vi "AutoSequencer.vi"(2 "Reinit Sequencer":bool, 7 "Auto Cluster In":T1) -> (8 "Auto Cluster Out":T1)   [LabVIEW 2020]
doc: "This VI manages the autonomous sequence. The drive base and manipulator sequencers operate in parallel. Autonomous plays are written as text files and uploaded to the roboRIO via FileZilla. The appropriate play is slected prior to the match via the FRC 4265 Dashboard. For each sequencer, each step is composed of a command and a parameter string of arbitrary length. Error checking and handling is supported. An autonomous test mode (for simulating autonomous plays on the robot cart) is supported. Status updates are sent to the FRC Driver Station and the FRC 4265 Dashboard throughout autonomous. Note that the autonomous sequencer may be also active during the begining of TeleOperated mode, as determined by the MasterRobotModeController.vi."
uses:
  GlobalPoseAndTargeting.vi
  GlobalDriverStationData.vi
  GlobalAutonomous.vi
panel:
  in  "Type Def":T1
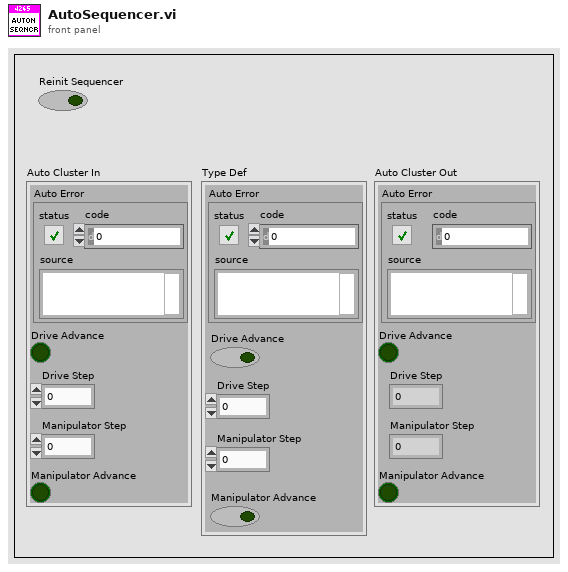
[diagram p1: front panel]
types:
  T1 = cluster{"Auto Error":errorcluster, "Drive Advance":bool, "Drive Step":i32, "Manipulator Step":i32, "Manipulator Advance":bool}
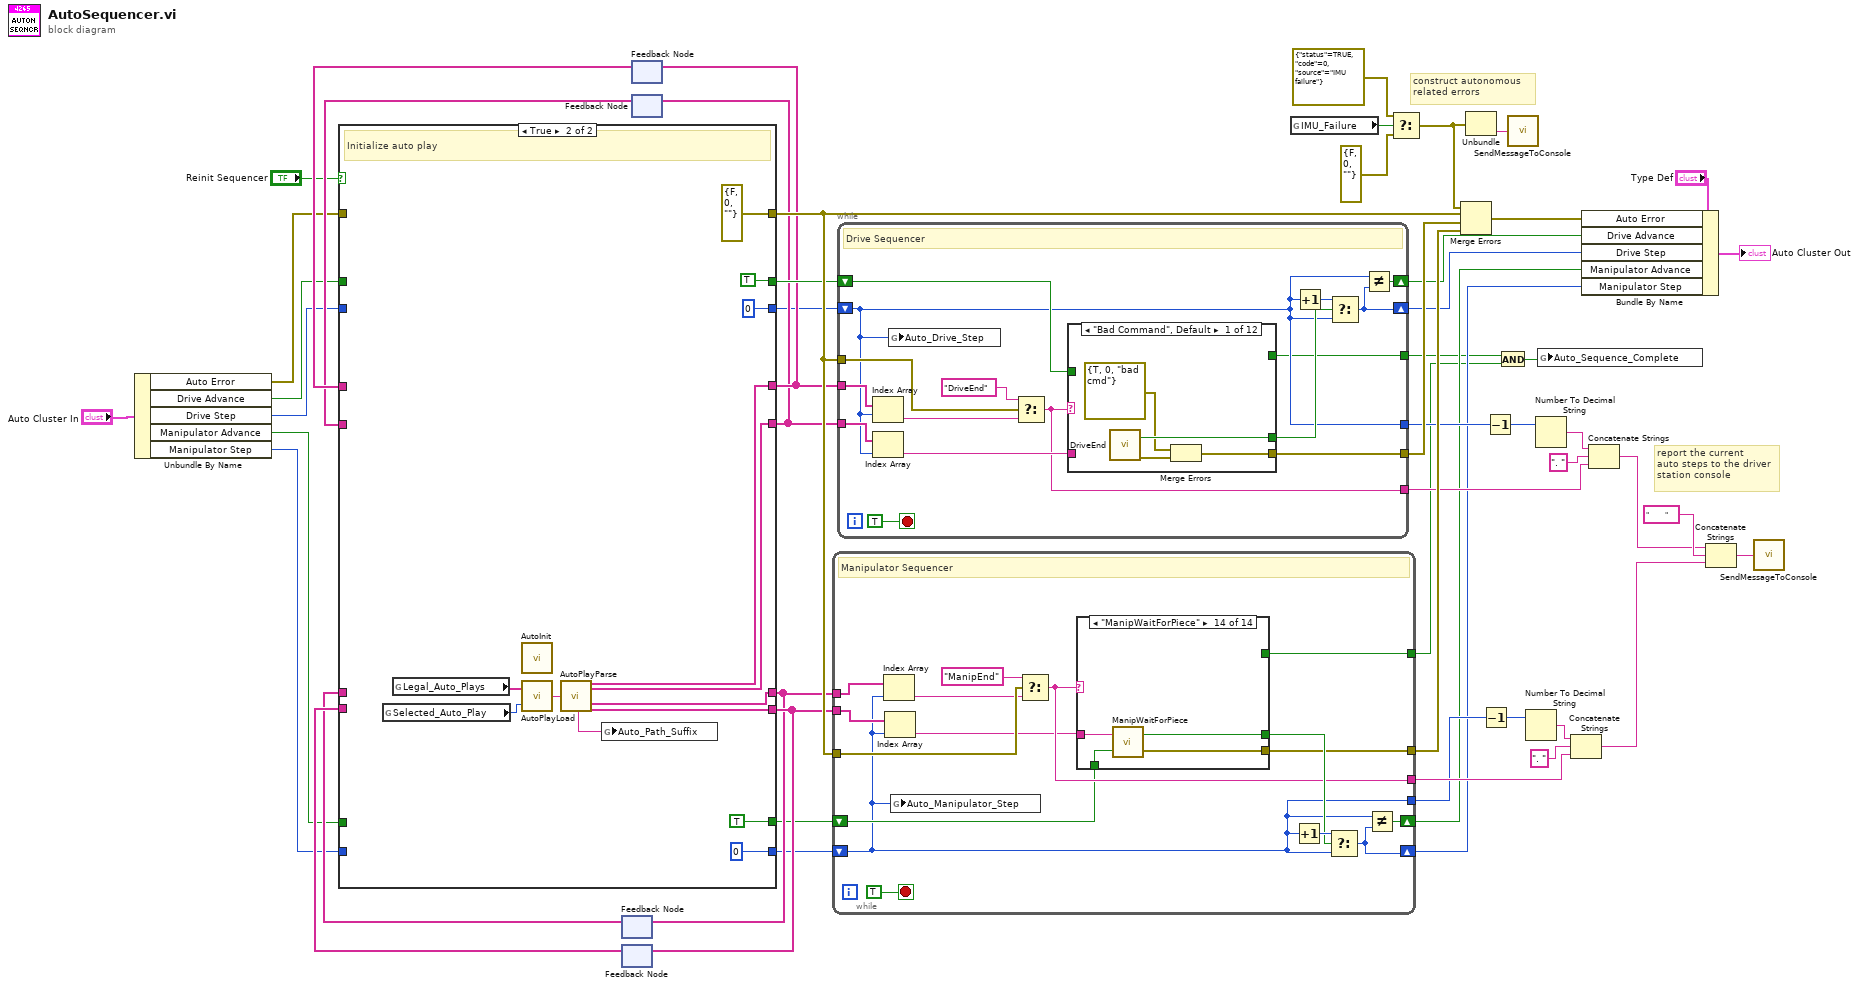
[diagram p0: block diagram]
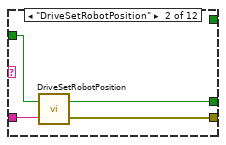
[diagram p2: hidden frame]
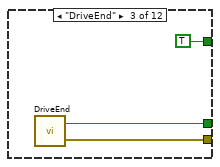
[diagram p3: hidden frame]
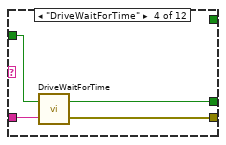
[diagram p4: hidden frame]
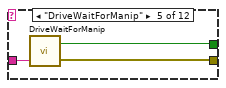
[diagram p5: hidden frame]
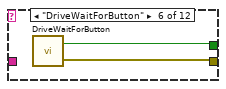
[diagram p6: hidden frame]
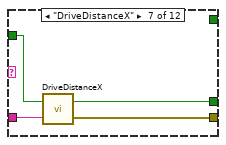
[diagram p7: hidden frame]
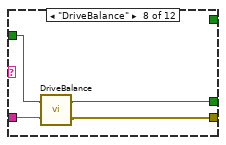
[diagram p8: hidden frame]
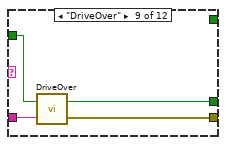
[diagram p9: hidden frame]
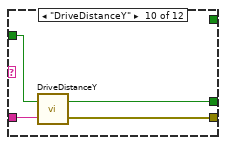
[diagram p10: hidden frame]
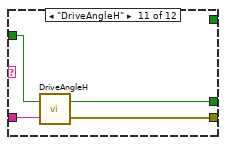
[diagram p11: hidden frame]
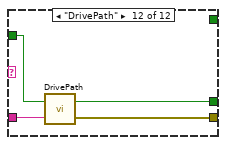
[diagram p12: hidden frame]
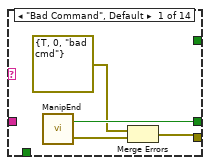
[diagram p14: hidden frame]
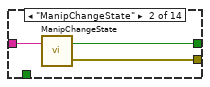
[diagram p15: hidden frame]
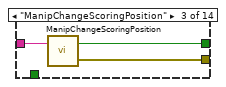
[diagram p16: hidden frame]
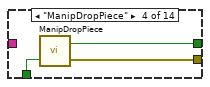
[diagram p17: hidden frame]
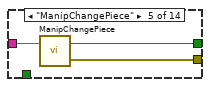
[diagram p18: hidden frame]
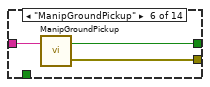
[diagram p19: hidden frame]
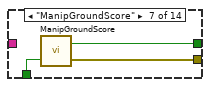
[diagram p20: hidden frame]
diagram:
  # "construct autonomous\nrelated errors"
  # "report the current\nauto steps to the driver\nstation console"
  n1 = Unbundle By Name("Auto Cluster In") -> ("Auto Error"=w11:errorcluster, "Drive Advance"=w10:bool, "Drive Step"=w9:i32, "Manipulator Advance"=w8:bool, "Manipulator Step"=w7:i32)
  n2 = feedback #1() -> (w41:string[])  [unwired: 1 in]
  n3 = feedback #2() -> (w42:string[])  [unwired: 1 in]
  n4 = feedback #3() -> (w47:string[])  [unwired: 1 in]
  n5 = feedback #4() -> (w46:string[])  [unwired: 1 in]
  n6 = case shown="True" "Reinit Sequencer" {
    tunnel: w7 -> [w59 _]
    tunnel: w8 -> [w60 _]
    tunnel: [w60 TRUE ("Advance Trigger")] -> w28
    tunnel: [w59 0] -> w37
    tunnel: [w58 w67] -> w39
    tunnel: [w57 w71] -> w40
    tunnel: w41 -> [w58 _]
    tunnel: w42 -> [w57 _]
    tunnel: [w56 0] -> w43
    tunnel: w9 -> [w56 _]
    tunnel: [w55 w69] -> w44
    tunnel: [w54 w68] -> w45
    tunnel: w46 -> [w55 _]
    tunnel: w47 -> [w54 _]
    tunnel: [w53 TRUE] -> w48
    tunnel: w10 -> [w53 _]
    tunnel: [w52 errorcluster {"status"=FALSE, "code"=0, "source"=""} ("error constant")] -> w50
    tunnel: w11 -> [w52 _]
    frame False {
      # "Continue auto play"
    }
    frame True {
      # "Initialize auto play"
      n7 = global read "GlobalDriverStationData.vi" "Selected_Auto_Play"() -> (w65:u16)
      n8 = global read "GlobalAutonomous.vi" "Legal_Auto_Plays"() -> (w63:string[])
      n9 = call "AutoInit.vi"() -> ()  [unwired: 1 in]
      n10 = call "AutoPlayLoad.vi"("Selected Auto Play"=w65, "Available Auto Plays"=w63) -> ("Loaded Auto Play"=w62:string)
      n11 = call "AutoPlayParse.vi"("Loaded Auto Play"=w62) -> ("Autonomous Path Suffix"=w61:string, "Drive Command Strings"=w68:string[], "Drive Parameter Strings"=w69:string[], "Manipulator Command Strings"=w67:string[], "Manipulator Parameter Strings"=w71:string[])  [unwired: 10 in, 4 out]
      n12 = global write "GlobalAutonomous.vi" "Auto_Path_Suffix"(w61) -> ()
    }
  }
  n13 = feedback-in #1(w39) -> ()
  n14 = feedback-in #2(w40) -> ()
  n15 = feedback-in #3(w45) -> ()
  n16 = feedback-in #4(w44) -> ()
  n17 = while {
    tunnel: w39 -> [w85]
    shift-right: [w87] -> w14
    shift-left: w37 -> [w75]
    shift-right: [w86] -> w15
    shift-left: w28 -> [w77]
    tunnel: w40 -> [w84]
    tunnel: [w79] -> w31
    tunnel: [w80] -> w51
    tunnel: w50 -> [w82]
    tunnel: [w75] -> w22
    tunnel: [w74] -> w4
    stop <- TRUE stop-if-true
    # "Manipulator Sequencer"
    n18 = Index Array(array=w85, index=w75) -> (element=w76:string)
    n19 = Index Array(array=w84, index=w75) -> (element=w78:string)
    n20 = global write "GlobalAutonomous.vi" "Auto_Manipulator_Step"(w75) -> ()
    n21 = Select(t="ManipEnd", s=w82, f=w76) -> (s? t:f=w79:string)
    n22 = case shown="\"ManipWaitForPiece\"" w79 {
      tunnel: w78 -> [_ w96 w99 _ w105 w108 _ _ _ w121 w124 _ w130 w134]
      tunnel: [w93 w95 w98 w101 w104 w107 w109 w114 w117 w119 w123 w126 w128 w131] -> w81
      tunnel: [w91 w94 w97 w100 w103 w106 w110 w113 w116 w118 w122 w125 w127 w132] -> w80
      tunnel: w77 -> [_ _ _ w102 _ _ w111 w112 _ w120 _ _ w129 w133]
      tunnel: [_ _ _ _ _ _ _ _ TRUE _ _ _ _ _] -> w74
      frame "Bad Command", Default {
        n23 = call "ManipEnd.vi"() -> ("Error Out"=w92:errorcluster, "Advance Trigger"=w93:bool)  [unwired: 2 in]
        n24 = Merge Errors(errorcluster {"status"=TRUE, "code"=0, "source"="bad cmd"} ("Path Follow Error"), w92) -> (w91:errorcluster)
      }
      frame "ManipChangeState" {
        n25 = call "ManipChangeState.vi"("Instruction String"=w96) -> ("Error Out"=w94:errorcluster, "Advance Trigger"=w95:bool)  [unwired: 1 in]
      }
      frame "ManipChangeScoringPosition" {
        n26 = call "ManipChangeScoringPosition.vi"("Instruction String"=w99) -> ("Error Out"=w97:errorcluster, "Advance Trigger"=w98:bool)  [unwired: 1 in]
      }
      frame "ManipDropPiece" {
        n27 = call "ManipDropPiece.vi"("Reinit"=w102) -> ("error out"=w100:errorcluster, "Advance Trigger"=w101:bool)  [unwired: 1 in]
      }
      frame "ManipChangePiece" {
        n28 = call "ManipChangePiece.vi"("Parameter String"=w105) -> ("error out"=w103:errorcluster, "Advance Trigger"=w104:bool)  [unwired: 1 in]
      }
      frame "ManipGroundPickup" {
        n29 = call "ManipGroundPickup.vi"("Parameter String"=w108) -> ("error out"=w106:errorcluster, "Advance Trigger"=w107:bool)  [unwired: 1 in]
      }
      frame "ManipGroundScore" {
        n30 = call "ManipGroundScore.vi"("Reinit"=w111) -> ("error out"=w110:errorcluster, "Advance Trigger"=w109:bool)  [unwired: 1 in]
      }
      frame "ManipWaitForArm" {
        n31 = call "ManipWaitForArm.vi"("Reint"=w112) -> ("error out"=w113:errorcluster, "Increment"=w114:bool)  [unwired: 1 in]
      }
      frame "ManipEnd" {
        n32 = call "ManipEnd.vi"() -> ("Error Out"=w116:errorcluster, "Advance Trigger"=w117:bool)  [unwired: 2 in]
      }
      frame "ManipWaitForTime" {
        n33 = call "ManipWaitForTime.vi"("Reinit"=w120, "Parameter String"=w121) -> ("Error Out"=w118:errorcluster, "Increment"=w119:bool)
      }
      frame "ManipWaitForDrive" {
        n34 = call "ManipWaitForDrive.vi"("Parameter String"=w124) -> ("Error Out"=w122:errorcluster, "Increment"=w123:bool)  [unwired: 1 in]
      }
      frame "ManipWaitForButton" {
        n35 = call "ManipWaitForButton.vi"() -> ("Error Out"=w125:errorcluster, "Increment"=w126:bool)  [unwired: 2 in]
      }
      frame "ManipWaitForDistance" {
        n36 = call "ManipWaitForDistance.vi"("Reinit"=w129, "Parameter String"=w130) -> ("Error Out"=w127:errorcluster, "Increment"=w128:bool)
      }
      frame "ManipWaitForPiece" {
        n37 = call "ManipWaitForPiece.vi"("Reinit"=w133, "Parameter String"=w134) -> ("Error Out"=w132:errorcluster, "Increment"=w131:bool)
      }
    }
    n38 = Increment(x=w75) -> (x+1=w89:i32)
    n39 = Select(t=w89, s=w81, f=w75) -> (s? t:f=w87:i32)
    n40 = Not Equal?(x=w75, y=w87) -> (x != y?=w86:bool)
  }
  n41 = while {
    shift-right: [w145] -> w16
    shift-left: w43 -> [w136]
    tunnel: w45 -> [w148]
    tunnel: w44 -> [w147]
    shift-right: [w144] -> w17
    shift-left: w48 -> [w143]
    tunnel: [w137] -> w36
    tunnel: w50 -> [w141]
    tunnel: [w138] -> w49
    tunnel: [w136] -> w23
    tunnel: [w135] -> w5
    stop <- TRUE stop-if-true
    # "Drive Sequencer"
    n42 = Index Array(array=w148, index=w136) -> (element=w140:string)
    n43 = Index Array(array=w147, index=w136) -> (element=w146:string)
    n44 = global write "GlobalAutonomous.vi" "Auto_Drive_Step"(w136) -> ()
    n45 = Select(t="DriveEnd", s=w141, f=w140) -> (s? t:f=w137:string)
    n46 = case shown="\"Bad Command\", Default" w137 {
      tunnel: w146 -> [_ w157 _ w163 w168 _ w173 w177 w179 w184 w188 w193]
      tunnel: [w154 w158 w161 w164 w166 w170 w172 w176 w181 w186 w190 w191] -> w142
      tunnel: w143 -> [_ w156 _ w162 _ _ w174 w178 w182 w185 w189 w194]
      tunnel: [w152 w155 w160 w165 w167 w169 w171 w175 w180 w183 w187 w192] -> w138
      tunnel: [_ _ TRUE _ _ _ _ _ _ _ _ _] -> w135
      frame "Bad Command", Default {
        n47 = call "DriveEnd.vi"() -> ("Error Out"=w153:errorcluster, "Advance Trigger"=w154:bool)  [unwired: 2 in]
        n48 = Merge Errors(errorcluster {"status"=TRUE, "code"=0, "source"="bad cmd"} ("Path Follow Error"), w153) -> (w152:errorcluster)
      }
      frame "DriveSetRobotPosition" {
        n49 = call "DriveSetRobotPosition.vi"("Parameter String"=w157, "Reinit"=w156) -> ("Error Out"=w155:errorcluster, "Increment"=w158:bool)
      }
      frame "DriveEnd" {
        n50 = call "DriveEnd.vi"() -> ("Error Out"=w160:errorcluster, "Advance Trigger"=w161:bool)  [unwired: 2 in]
      }
      frame "DriveWaitForTime" {
        n51 = call "DriveWaitForTime.vi"("Parameter String"=w163, "Reinit"=w162) -> ("Error Out"=w165:errorcluster, "Increment"=w164:bool)
      }
      frame "DriveWaitForManip" {
        n52 = call "DriveWaitForManip.vi"("Parameter String"=w168) -> ("Error Out"=w167:errorcluster, "Increment"=w166:bool)  [unwired: 1 in]
      }
      frame "DriveWaitForButton" {
        n53 = call "DriveWaitForButton.vi"() -> ("Error Out"=w169:errorcluster, "Increment"=w170:bool)  [unwired: 2 in]
      }
      frame "DriveDistanceX" {
        n54 = call "DriveDistanceX.vi"("Parameter String"=w173, "Reinit"=w174) -> ("Error Out"=w171:errorcluster, "Increment"=w172:bool)
      }
      frame "DriveBalance" {
        n55 = call "DriveBalance.vi"("Parameter String"=w177, "Reinit"=w178) -> ("Error Out"=w175:errorcluster, "Increment"=w176:bool)
      }
      frame "DriveOver" {
        n56 = call "DriveOver.vi"("Parameter String"=w179, "Reinit"=w182) -> ("Error Out"=w180:errorcluster, "Increment"=w181:bool)
      }
      frame "DriveDistanceY" {
        n57 = call "DriveDistanceY.vi"("Parameter String"=w184, "Reinit"=w185) -> ("Error Out"=w183:errorcluster, "Increment"=w186:bool)
      }
      frame "DriveAngleH" {
        n58 = call "DriveAngleH.vi"("Parameter String"=w188, "Reinit"=w189) -> ("Error Out"=w187:errorcluster, "Increment"=w190:bool)
      }
      frame "DrivePath" {
        n59 = call "DrivePath.vi"("Parameter String"=w193, "Reinit"=w194) -> ("Path Follower Error"=w192:errorcluster, "Increment"=w191:bool)
      }
    }
    n60 = Increment(x=w136) -> (x+1=w149:i32)
    n61 = Select(t=w149, s=w142, f=w136) -> (s? t:f=w145:i32)
    n62 = Not Equal?(x=w136, y=w145) -> (x != y?=w144:bool)
  }
  n63 = global read "GlobalPoseAndTargeting.vi" "IMU_Failure"() -> (w19:bool)
  n64 = Select(t=errorcluster {"status"=TRUE, "code"=0, "source"="IMU failure"} ("error constant"), s=w19, f=errorcluster {"status"=FALSE, "code"=0, "source"=""} ("error constant")) -> (s? t:f=w21:errorcluster)
  n65 = Merge Errors(w21, w50, w49, w51) -> (w18:errorcluster)
  n66 = Unbundle(w21) -> ("source"=w20:string)  [unwired: 2 out]
  n67 = Decrement(x=w22) -> (x-1=w1:i32)
  n68 = Decrement(x=w23) -> (x-1=w2:i32)
  n69 = And(x=w5, y=w4) -> (x .and. y?=w6:bool)
  n70 = call "SendMessageToConsole.vi"("Message String"=w20) -> ()  [unwired: 1 in]
  n71 = Number To Decimal String(number=w1) -> (decimal integer string=w32:string)  [unwired: 1 in]
  n72 = Number To Decimal String(number=w2) -> (decimal integer string=w34:string)  [unwired: 1 in]
  n73 = global write "GlobalAutonomous.vi" "Auto_Sequence_Complete"(w6) -> ()
  n74 = Concatenate Strings(w32, ". " ("string"), w31) -> (w25:string)
  n75 = Bundle By Name(cluster="Type Def", "Auto Error"=w18, "Drive Advance"=w17, "Drive Step"=w16, "Manipulator Advance"=w15, "Manipulator Step"=w14) -> (→"Auto Cluster Out":T1)
  n76 = Concatenate Strings(w34, ". " ("string"), w36) -> (w26:string)
  n77 = Concatenate Strings(w26, "        " ("string"), w25) -> (w24:string)
  n78 = call "SendMessageToConsole.vi"("Message String"=w24) -> ()  [unwired: 1 in]
